vi "E07_Formula_Not.vi"() -> ()   [LabVIEW 2026]
panel:
  out "Numeric 2":dbl
  out "Numeric":dbl
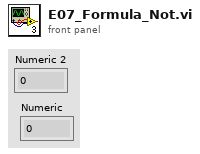
[diagram p1: front panel]
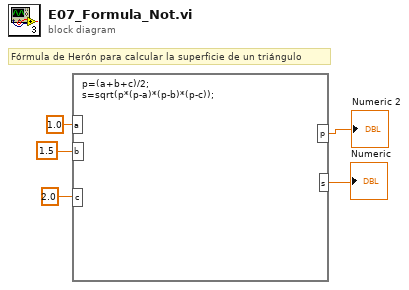
[diagram p0: block diagram]
diagram:
  # "Fórmula de Herón para calcular la superficie de un triángulo"
  n1 = formula code="p=(a+b+c)/2;\ns=sqrt(p*(p-a)*(p-b)*(p-c));"("a"=1.0 ("input variable"), "b"=1.5 ("input variable"), "c"=2.0 ("input variable")) -> ("p"=→"Numeric 2":dbl, "s"=→"Numeric":dbl)
